vi "laneleftright412_temp.vi"() -> ()   [LabVIEW 2015]
uses:
  <vilib>/Analysis/1siggen.llb/Ramp Pattern by Delta.vi
  G_ALL.vi
  <vilib>/Analysis/polynomials.llb/nth Derivative of Polynomial (DBL).vi
  <vilib>/Analysis/polynomials.llb/Scalar Polynomial Evaluation (DBL).vi
  G_LCM.vi
  G_SEN.vi
  <vilib>/Analysis/NI_AALBase.lvlib
  <vilib>/Analysis/NI_AALPro.lvlib
panel:
  out "size(s)":i32
  out "lf_shift":dbl
  out "lr_shift":dbl
  out "rf_shift":dbl
  out "rr_shift":dbl
  in  "gain":dbl=1.0
  out "y_shift":dbl format="%#_13g"
  out "x_shift":dbl format="%#_13g"
  in  "d_safe":dbl=0.4
  out "R0":dbl
  out "y_ramp":dbl[](array[numeric])
  out "y_car":dbl[](array[numeric])
  out "x_car":dbl[](array[numeric])
  out "x_rf":dbl[](array[numeric])
  out "y_rf":dbl[](array[numeric])
  out "y_rr":dbl[](array[numeric])
  out "x_rr":dbl[](array[numeric])
  out "x_lr":dbl[](array[numeric])
  out "y_lr":dbl[](array[numeric])
  out "af":dbl
  out "y_lf":dbl[](array[numeric])
  out "x_lf":dbl[](array[numeric])
  out "h_path":dbl[](array[numeric])
  out "x_path":dbl[](array[numeric])
  out "y_path":dbl[](array[numeric])
  out "gap":dbl
  out "theta":dbl[](array[numeric])
  out "y":dbl[](array[numeric])
  out "x":dbl[](array[numeric])
  out "r":dbl[](array[numeric])
  out "rout":dbl[](array[numeric])
  out "rin":dbl[](array[numeric])
  out "XY Graph":cluster{"Y":dbl[], "Y":dbl[]}[](graph)
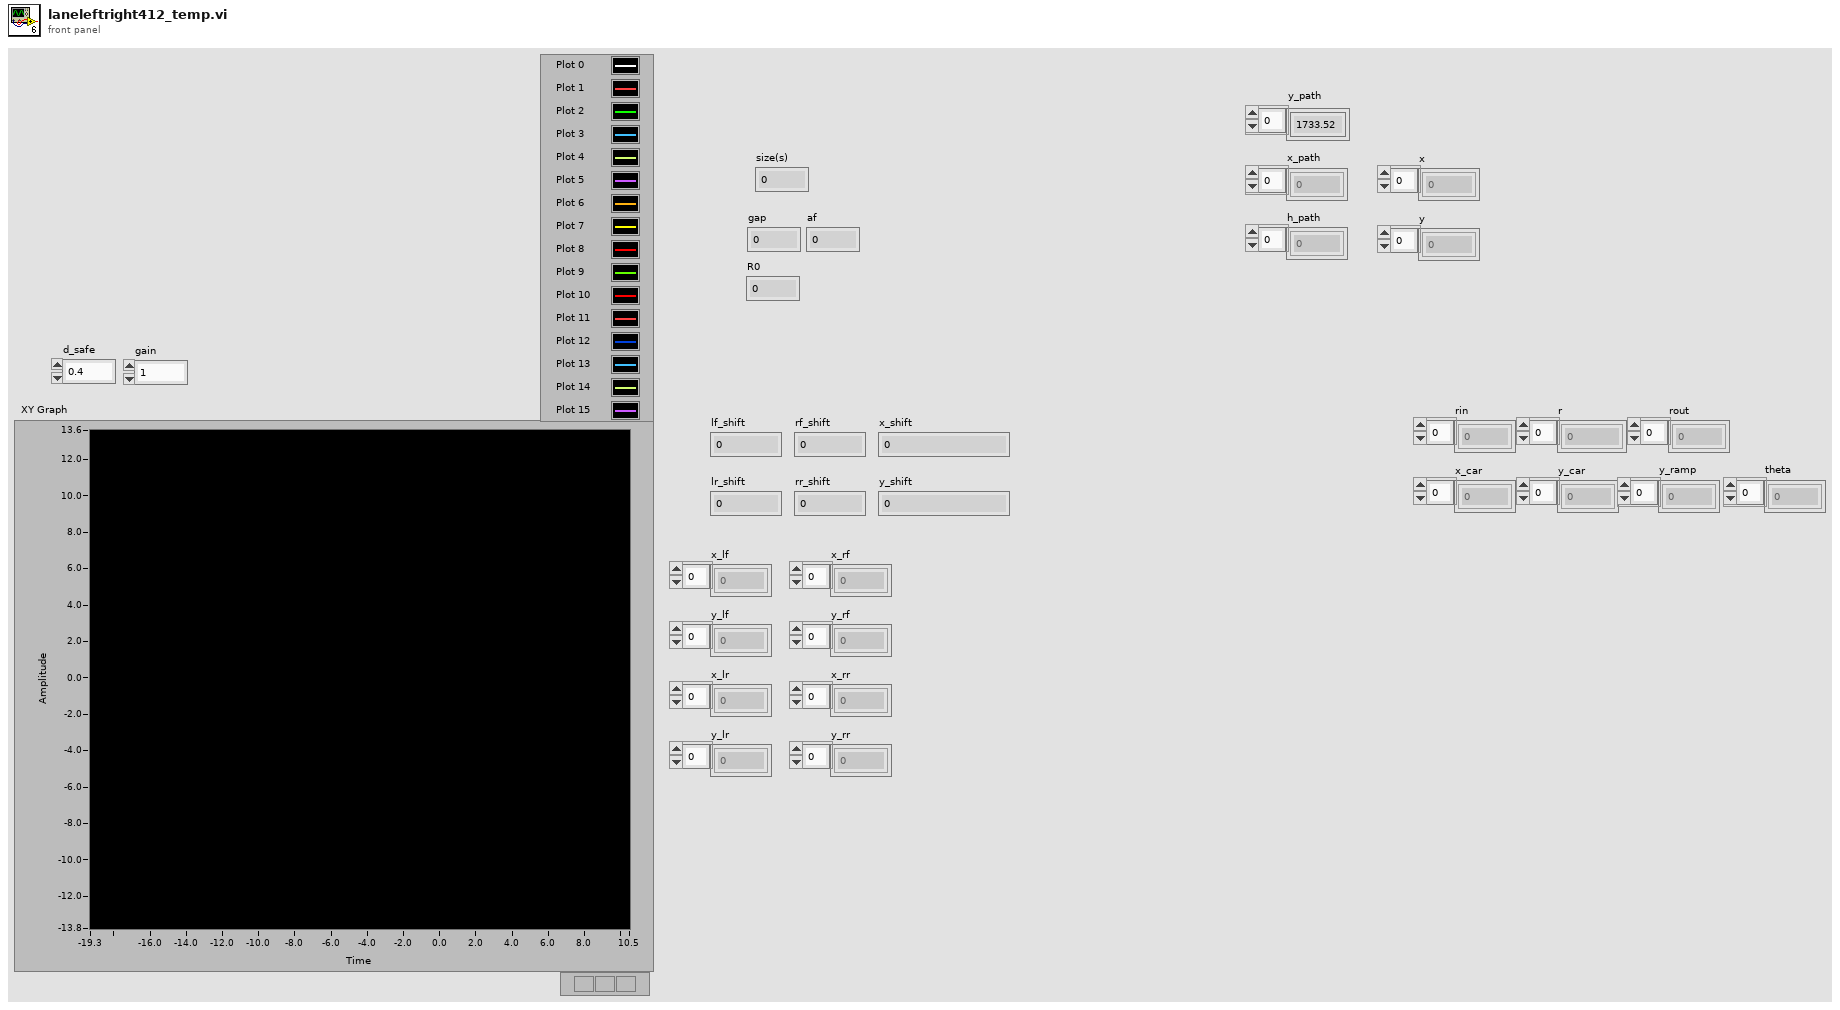
[diagram p1: front panel]
types:
  T1 = cluster{"C_Wheel base":dbl, "ratio_steer":dbl, "Overall width":dbl, "af":dbl, "turn radius":dbl, "eval":dbl, "ap":dbl, "an":dbl, "Vmax":dbl, "mu":dbl, "Vlast":dbl}
  T2 = cluster{"hash":i64, "sys time":i64, "size":i64, "x":dbl[], "y":dbl[], "point_flag":i32[]}
  T3 = cluster{"delta":bool, "Rotational position":dbl, "Rotational position":dbl}[]
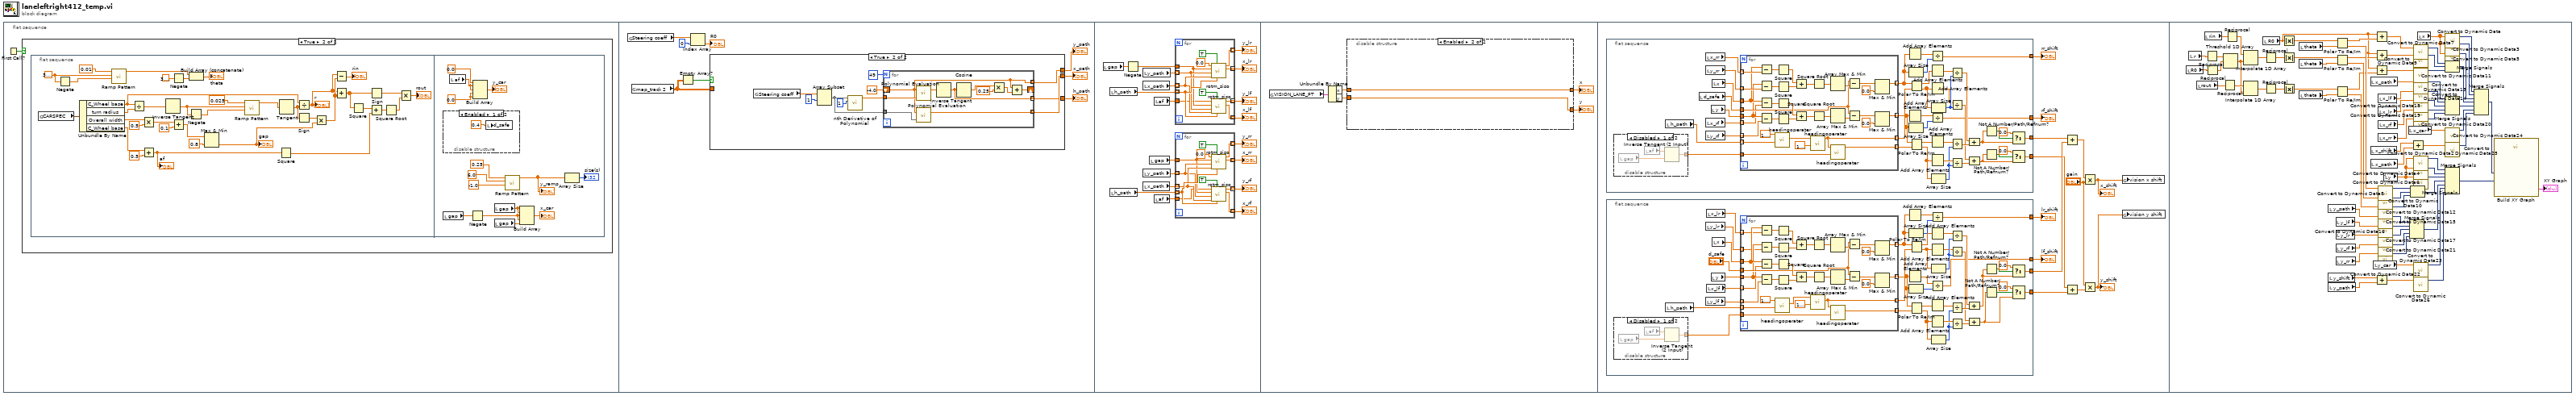
[diagram p0: block diagram]
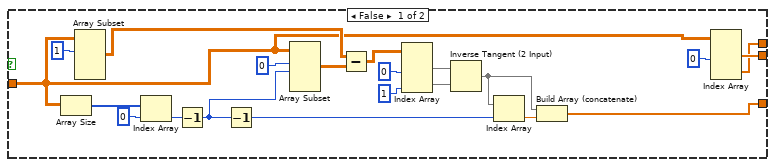
[diagram p4: hidden frame]
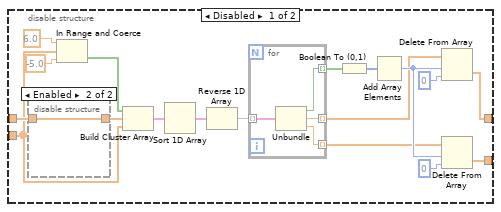
[diagram p5: hidden frame]
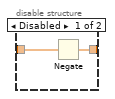
[diagram p6: hidden frame]
diagram:
  n1 = flat-sequence {
    frame #0 {
      n2 = First Call?() -> (First Call?: T/F=w1:bool)
      n3 = case shown="True" w1 {
        frame False {
        }
        frame True {
          n4 = flat-sequence {
            frame #0 {
              w20 = 3.141592653589793
              n5 = global read "G_ALL.vi" "CARSPEC"() -> (w38:T1)
              n6 = Negate(x=w20) -> (-x=w21:dbl)
              n7 = Unbundle By Name(w38) -> ("C_Wheel base"=w18:dbl, "turn radius"=w37:dbl, "Overall width"=w32:dbl, "C_Wheel base"=w4:dbl)
              n8 = call-poly <vilib>:"Ramp Pattern.vi"("start"=w21, "end"=w20, "delta"=0.01) -> ("Ramp Pattern"=w15:dbl[])  [unwired: 6 in, 2 out]
              n9 = Divide(x=w18, y=w37) -> (x/y=w36:dbl)
              n10 = Multiply(x=w32, y=0.5) -> (x*y=w17:dbl)
              n11 = Add(x=w4, y=0.5) -> (x+y=w2:dbl)
              "af" <- w2
              n12 = Inverse Tangent(1:w36) -> (0:w35:dbl)
              n13 = Negate(x=3.141592653589793) -> (-x=w12:dbl)
              n14 = Add(x=w17, y=0.1) -> (x+y=w7:dbl)
              n15 = Negate(x=w35) -> (-x=w8:dbl)
              n16 = Build Array (concatenate)(w15, w12) -> (→"theta":dbl[])
              n17 = Max & Min(x=w7, y=0.8) -> (min(x,y)=w6:dbl)  [unwired: 1 out]
              "gap" <- w6
              n18 = call-poly <vilib>:"Ramp Pattern.vi"("start"=w8, "end"=w35, "delta"=0.025) -> ("Ramp Pattern"=w33:dbl[])  [unwired: 6 in, 2 out]
              n19 = Square(x=w2) -> (x^2=w26:dbl)
              n20 = Tangent(1:w33) -> (0:w30:dbl[])
              n21 = Divide(x=w18, y=w30) -> (x/y=w11:dbl[])
              "r" <- w11
              n22 = Sign(1:w30) -> (0:w29:dbl[])
              n23 = Multiply(x=w29, y=w6) -> (x*y=w28:dbl[])
              n24 = Subtract(x=w11, y=w28) -> (x-y=→"rin":dbl[])
              n25 = Add(x=w11, y=w28) -> (x+y=w24:dbl[])
              n26 = Square(x=w24) -> (x^2=w27:dbl[])
              n27 = Sign(1:w24) -> (0:w22:dbl[])
              n28 = Add(x=w27, y=w26) -> (x+y=w25:dbl[])
              n29 = Square Root(x=w25) -> (sqrt(x)=w23:dbl[])
              n30 = Multiply(x=w22, y=w23) -> (x*y=→"rout":dbl[])
            }
            frame #1 {
              w45 = 0.0 ("element")
              n31 = disable-structure shown="Enabled" {
                frame Enabled {
                  n32 = local write "d_safe"(0.4 ("d_safe")) -> ()
                }
                frame Disabled {
                }
              }
              n33 = local read "gap"() -> (w52:dbl)
              n34 = local read "af"() -> (w47:dbl)
              n35 = Negate(x=w52) -> (-x=w50:dbl)
              n36 = Build Array(0.0 ("element"), w47, w47, w45, w45) -> (→"y_car":dbl[])
              n37 = local read "gap"() -> (w51:dbl)
              n38 = local read "gap"() -> (w49:dbl)
              n39 = call-poly <vilib>:"Ramp Pattern.vi"("start"=-1.0, "end"=6.0, "delta"=0.25) -> ("Ramp Pattern"=w40:dbl[])  [unwired: 6 in, 2 out]
              "y_ramp" <- w40
              n40 = Build Array(w51, w51, w50, w50, w49) -> (→"x_car":dbl[])
              n41 = Array Size(array=w40) -> (size(s)=→"size(s)":i32)
            }
          }
        }
      }
    }
    frame #1 {
      n42 = global read "G_ALL.vi" "Steering coeff"() -> (w58:dbl[])
      n43 = global read "G_ALL.vi" "map_track 2"() -> (w54:dbl[][])
      n44 = Empty Array?(array=w54) -> (empty?=w55:bool)
      n45 = Index Array(array=w58, index=0) -> (element=→"R0":dbl)
      n46 = case shown="True" w55 {
        tunnel: [w82 w92] -> w61
        tunnel: [w81 w90] -> w60
        tunnel: [w80 w91] -> w59
        tunnel: w54 -> [w62 _]
        frame False {
          n47 = Array Size(array=w62) -> (size(s)=w77:i32[])
          n48 = Array Subset(array=w62, index (row)=1 ("index")) -> (w73:dbl[][])  [unwired: 3 in]
          n49 = Index Array(array=w77, index=0) -> (element=w75:i32)
          n50 = Decrement(x=w75) -> (x-1=w67:i32)
          n51 = Decrement(x=w67) -> (x-1=w66:i32)
          n52 = Array Subset(array=w62, index (row)=0 ("index"), length (row)=w67) -> (w74:dbl[][])  [unwired: 2 in]
          n53 = Subtract(x=w73, y=w74) -> (x-y=w72:dbl[][])
          n54 = Index Array(array=w72, index (col) #1=0 ("disabled index (col)"), index (col) #2=1 ("index (col)")) -> (element #1=w69:dbl[], element #2=w68:dbl[])  [unwired: 2 in]
          n55 = Inverse Tangent (2 Input)(1:w68, 2:w69) -> (0:w64:dbl[])
          n56 = Index Array(array=w64, index=w66) -> (element=w65:dbl)
          n57 = Build Array (concatenate)(w64, w65) -> (w81:dbl[])
          n58 = Index Array(array=w62, index (col) #1=0 ("disabled index (col)")) -> (element #1=w82:dbl[], element #2=w80:dbl[])  [unwired: 3 in]
        }
        frame True {
          n59 = global read "G_ALL.vi" "Steering coeff"() -> (w83:dbl[])
          n60 = Array Subset(array=w83, index=1) -> (w85:dbl[])  [unwired: 1 in]
          n61 = call-poly <vilib>:"nth Derivative of Polynomial.vi"("order"=1, "P(x)"=w85) -> ("Nth Derivative of P(x)"=w86:dbl[])  [unwired: 8 in, 1 out]
          n62 = for {
            N: 49 -> [_]
            shift-right: [w93] -> _
            shift-left: -4.0 -> [w94]
            tunnel: w86 -> [w102]
            tunnel: w85 -> [w98]
            tunnel: [w97] -> w92 mode=indexing
            tunnel: [w94] -> w91 mode=indexing
            tunnel: [w96] -> w90 mode=indexing
            n63 = call-poly <vilib>:"Polynomial Evaluation.vi"("P(x)"=w102, "a"=w94) -> ("P(a)"=w101:dbl)  [unwired: 1 out]
            n64 = call-poly <vilib>:"Polynomial Evaluation.vi"("P(x)"=w98, "a"=w94) -> ("P(a)"=w97:dbl)  [unwired: 1 out]
            n65 = Inverse Tangent(1:w101) -> (0:w96:dbl)
            n66 = Cosine(x=w96) -> (cos(x)=w100:dbl)
            n67 = Multiply(x=w100, y=0.25) -> (x*y=w95:dbl)
            n68 = Add(x=w94, y=w95) -> (x+y=w93:dbl)
          }
        }
      }
      "y_path" <- w59
      "x_path" <- w61
      "h_path" <- w60
    }
    frame #2 {
      n69 = local read "gap"() -> (w118:dbl)
      n70 = local read "h_path"() -> (w119:dbl[])
      n71 = local read "h_path"() -> (w108:dbl[])
      n72 = Negate(x=w118) -> (-x=w117:dbl)
      n73 = local read "y_path"() -> (w120:dbl[])
      n74 = local read "x_path"() -> (w121:dbl[])
      n75 = local read "y_path"() -> (w107:dbl[])
      n76 = local read "x_path"() -> (w106:dbl[])
      n77 = local read "gap"() -> (w105:dbl)
      n78 = local read "af"() -> (w104:dbl)
      n79 = local read "af"() -> (w103:dbl)
      n80 = for {
        tunnel: w121 -> [w141] mode=indexing
        tunnel: w120 -> [w140] mode=indexing
        tunnel: w119 -> [w142] mode=indexing
        tunnel: [w145] -> w116 mode=indexing
        tunnel: [w144] -> w115 mode=indexing
        tunnel: w117 -> [w139]
        tunnel: [w137] -> w114 mode=indexing
        tunnel: [w136] -> w113 mode=indexing
        tunnel: w104 -> [w134]
        n81 = call "rotm_siso.vi"("angle[rad]"=w142, "reverse"=TRUE, "y0"=w141, "x0"=w140, "y"=w139, "x"=0.0) -> ("y'"=w136:dbl, "x'"=w137:dbl)  [unwired: 4 in]
        n82 = call "rotm_siso.vi"("angle[rad]"=w142, "reverse"=TRUE, "y0"=w141, "x0"=w140, "y"=w139, "x"=w134) -> ("y'"=w144:dbl, "x'"=w145:dbl)  [unwired: 4 in]
      }
      "x_lf" <- w115
      "y_lf" <- w116
      "y_lr" <- w114
      "x_lr" <- w113
      n83 = for {
        tunnel: w106 -> [w129] mode=indexing
        tunnel: w107 -> [w128] mode=indexing
        tunnel: w108 -> [w130] mode=indexing
        tunnel: [w133] -> w109 mode=indexing
        tunnel: [w132] -> w110 mode=indexing
        tunnel: w105 -> [w123]
        tunnel: [w126] -> w111 mode=indexing
        tunnel: [w125] -> w112 mode=indexing
        tunnel: w103 -> [w122]
        n84 = call "rotm_siso.vi"("angle[rad]"=w130, "reverse"=TRUE, "y0"=w129, "x0"=w128, "y"=w123, "x"=0.0) -> ("y'"=w125:dbl, "x'"=w126:dbl)  [unwired: 4 in]
        n85 = call "rotm_siso.vi"("angle[rad]"=w130, "reverse"=TRUE, "y0"=w129, "x0"=w128, "y"=w123, "x"=w122) -> ("y'"=w132:dbl, "x'"=w133:dbl)  [unwired: 4 in]
      }
      "x_rf" <- w110
      "y_rf" <- w109
      "y_rr" <- w111
      "x_rr" <- w112
    }
    frame #3 {
      n86 = global read "G_LCM.vi" "VISION_LANE_PT"() -> (w150:T2)
      n87 = Unbundle By Name(w150) -> ("x"=w149:dbl[], "y"=w148:dbl[])
      n88 = disable-structure shown="Enabled" {
        disable-tunnel: w149 -> [w167 w177]
        disable-tunnel: [w165 w176] -> w146
        disable-tunnel: [w164 w177] -> w147
        disable-tunnel: w148 -> [w161 w176]
        frame Disabled {
          n89 = disable-structure shown="Enabled" {
            disable-tunnel: w167 -> [w170 w171]
            disable-tunnel: [w169 w171] -> w168
            frame Disabled {
              n90 = Negate(x=w170) -> (-x=w169:dbl[])
            }
            frame Enabled {
            }
          }
          n91 = In Range and Coerce(upper limit=6.0 ("delta"), x=w161, lower limit=-5.0) -> (In Range?=w159:bool[])  [unwired: 1 out]
          n92 = Build Cluster Array(w159, w168, w161) -> (w157:T3)
          n93 = Sort 1D Array(array=w157) -> (sorted array=w158:T3)
          n94 = Reverse 1D Array(array=w158) -> (reversed array=w154:T3)
          n95 = for {
            tunnel: w154 -> [w175] mode=indexing
            tunnel: [w174] -> w152 mode=indexing
            tunnel: [w173] -> w151 mode=indexing
            tunnel: [w172] -> w162 mode=indexing
            n96 = Unbundle(w175) -> ("delta"=w172:bool, "Rotational position"=w174:dbl, "Rotational position"=w173:dbl)
          }
          n97 = Boolean To (0,1)(Boolean=w162) -> (0, 1=w155:i16[])
          n98 = Add Array Elements(numeric array=w155) -> (sum=w163:i16)
          n99 = Delete From Array(array=w152, length=w163, index=0) -> (deleted portion=w164:dbl[])  [unwired: 1 out]
          n100 = Delete From Array(array=w151, length=w163, index=0) -> (deleted portion=w165:dbl[])  [unwired: 1 out]
        }
        frame Enabled {
        }
      }
      "x" <- w147
      "y" <- w146
    }
    frame #4 {
      n101 = flat-sequence {
        tunnel: [w203] -> w180
        tunnel: [w202] -> w183
        tunnel: [w196] -> w185
        tunnel: [w195] -> w184
        frame #0 {
          n102 = disable-structure shown="Disabled" {
            disable-tunnel: [w233 _] -> w194
            frame Disabled {
              n103 = local read "gap"() -> (w234:dbl)
              n104 = local read "af"() -> (w232:dbl)
              n105 = Inverse Tangent (2 Input)(1:w234, 2:w232) -> (0:w233:dbl)
            }
            frame Enabled {
            }
          }
          n106 = local read "h_path"() -> (w227:dbl[])
          n107 = local read "d_safe"() -> (w191:dbl)
          n108 = local read "x_rr"() -> (w226:dbl[])
          n109 = local read "y_rr"() -> (w225:dbl[])
          n110 = local read "x_rf"() -> (w228:dbl[])
          n111 = local read "y_rf"() -> (w229:dbl[])
          n112 = local read "y"() -> (w230:dbl[])
          n113 = local read "x"() -> (w231:dbl[])
          n114 = for {
            tunnel: w231 -> [w245]
            tunnel: w230 -> [w244]
            tunnel: w229 -> [w268] mode=indexing
            tunnel: w228 -> [w240] mode=indexing
            tunnel: w227 -> [w242] mode=indexing
            tunnel: [w236] -> w224 mode=indexing
            tunnel: w191 -> [w246]
            tunnel: [w259] -> w192 mode=indexing
            tunnel: [w258] -> w199 mode=indexing
            tunnel: w226 -> [w248] mode=indexing
            tunnel: w225 -> [w247] mode=indexing
            tunnel: w194 -> [w235]
            tunnel: [w237] -> w193 mode=indexing
            n115 = Subtract(x=w245, y=w248) -> (x-y=w249:dbl[])
            n116 = Subtract(x=w244, y=w247) -> (x-y=w250:dbl[])
            n117 = Subtract(x=w245, y=w240) -> (x-y=w267:dbl[])
            n118 = Subtract(x=w244, y=w268) -> (x-y=w266:dbl[])
            n119 = call "headingoperater.vi"("h1"=w242, "h2"=1.5707963267948966) -> ("h2-h1"=w241:dbl)  [unwired: 8 in, 1 out]
            n120 = Square(x=w249) -> (x^2=w252:dbl[])
            n121 = Square(x=w250) -> (x^2=w251:dbl[])
            n122 = Square(x=w267) -> (x^2=w264:dbl[])
            n123 = Square(x=w266) -> (x^2=w265:dbl[])
            n124 = Add(x=w252, y=w251) -> (x+y=w253:dbl[])
            n125 = Add(x=w264, y=w265) -> (x+y=w263:dbl[])
            n126 = call "headingoperater.vi"("h1"=1.5707963267948966, "h2"=w241) -> ("h2+h1"=w236:dbl)  [unwired: 8 in, 1 out]
            n127 = Square Root(x=w253) -> (sqrt(x)=w254:dbl[])
            n128 = Square Root(x=w263) -> (sqrt(x)=w262:dbl[])
            n129 = Array Max & Min(array=w254) -> (min value=w255:dbl)  [unwired: 3 out]
            n130 = Array Max & Min(array=w262) -> (min value=w239:dbl)  [unwired: 3 out]
            n131 = call "headingoperater.vi"("h1"=w235, "h2"=w236) -> ("h2+h1"=w237:dbl)  [unwired: 8 in, 1 out]
            n132 = Subtract(x=w246, y=w255) -> (x-y=w256:dbl)
            n133 = Subtract(x=w246, y=w239) -> (x-y=w238:dbl)
            n134 = Max & Min(x=w256, y=0.0) -> (max(x,y)=w258:dbl)  [unwired: 1 out]
            n135 = Max & Min(x=w238, y=0.0) -> (max(x,y)=w259:dbl)  [unwired: 1 out]
          }
          n136 = Add Array Elements(numeric array=w199) -> (sum=w201:dbl)
          n137 = Add Array Elements(numeric array=w192) -> (sum=w197:dbl)
          n138 = Array Size(array=w199) -> (size(s)=w200:i32)
          n139 = Array Size(array=w192) -> (size(s)=w198:i32)
          n140 = Polar To Re/Im(2:w224, 3:w199) -> (0:w219:dbl[], 1:w220:dbl[])
          n141 = Polar To Re/Im(2:w193, 3:w192) -> (0:w214:dbl[], 1:w215:dbl[])
          n142 = Divide(x=w201, y=w200) -> (x/y=w196:dbl)
          n143 = Add Array Elements(numeric array=w220) -> (sum=w222:dbl)
          n144 = Add Array Elements(numeric array=w219) -> (sum=w221:dbl)
          n145 = Divide(x=w197, y=w198) -> (x/y=w195:dbl)
          n146 = Add Array Elements(numeric array=w215) -> (sum=w217:dbl)
          n147 = Add Array Elements(numeric array=w214) -> (sum=w218:dbl)
          n148 = Array Size(array=w219) -> (size(s)=w223:i32)
          n149 = Array Size(array=w214) -> (size(s)=w216:i32)
          n150 = Divide(x=w222, y=w223) -> (x/y=w213:dbl)
          n151 = Divide(x=w221, y=w223) -> (x/y=w211:dbl)
          n152 = Divide(x=w217, y=w216) -> (x/y=w212:dbl)
          n153 = Divide(x=w218, y=w216) -> (x/y=w210:dbl)
          n154 = Compound Arithmetic op=ADD(w213, w212) -> (w207:dbl)
          n155 = Compound Arithmetic op=ADD(w211, w210) -> (w204:dbl)
          n156 = Not A Number/Path/Refnum?(number/path/refnum=w207) -> (NaN/Path/Refnum?=w208:bool)
          n157 = Not A Number/Path/Refnum?(number/path/refnum=w204) -> (NaN/Path/Refnum?=w206:bool)
          n158 = Select(t=0.0, s=w208, f=w207) -> (s? t:f=w202:dbl)
          n159 = Select(t=0.0, s=w206, f=w204) -> (s? t:f=w203:dbl)
        }
      }
      n160 = flat-sequence {
        tunnel: [w280] -> w179
        tunnel: [w279] -> w182
        tunnel: [w272] -> w188
        tunnel: [w271] -> w187
        frame #0 {
          n161 = disable-structure shown="Disabled" {
            disable-tunnel: [w311 _] -> w270
            frame Disabled {
              n162 = local read "gap"() -> (w312:dbl)
              n163 = local read "af"() -> (w310:dbl)
              n164 = Inverse Tangent (2 Input)(1:w312, 2:w310) -> (0:w311:dbl)
            }
            frame Enabled {
            }
          }
          n165 = local read "h_path"() -> (w307:dbl[])
          n166 = local read "y_lr"() -> (w303:dbl[])
          n167 = local read "y_lf"() -> (w301:dbl[])
          n168 = local read "x_lr"() -> (w304:dbl[])
          n169 = local read "x_lf"() -> (w302:dbl[])
          n170 = local read "y"() -> (w308:dbl[])
          n171 = local read "x"() -> (w309:dbl[])
          n172 = for {
            tunnel: w309 -> [w324]
            tunnel: w308 -> [w323]
            tunnel: w307 -> [w317] mode=indexing
            tunnel: "d_safe" -> [w325]
            tunnel: [w315] -> w305 mode=indexing
            tunnel: [w336] -> w273 mode=indexing
            tunnel: [w337] -> w276 mode=indexing
            tunnel: w304 -> [w322] mode=indexing
            tunnel: w303 -> [w321] mode=indexing
            tunnel: w302 -> [w320] mode=indexing
            tunnel: w301 -> [w319] mode=indexing
            tunnel: w270 -> [w313]
            tunnel: [w314] -> w269 mode=indexing
            n173 = Subtract(x=w324, y=w322) -> (x-y=w346:dbl[])
            n174 = Subtract(x=w323, y=w321) -> (x-y=w345:dbl[])
            n175 = Subtract(x=w324, y=w320) -> (x-y=w326:dbl[])
            n176 = Subtract(x=w323, y=w319) -> (x-y=w327:dbl[])
            n177 = call "headingoperater.vi"("h1"=w317, "h2"=1.5707963267948966) -> ("h2-h1"=w316:dbl)  [unwired: 8 in, 1 out]
            n178 = Square(x=w346) -> (x^2=w343:dbl[])
            n179 = Square(x=w345) -> (x^2=w344:dbl[])
            n180 = Square(x=w326) -> (x^2=w329:dbl[])
            n181 = Square(x=w327) -> (x^2=w328:dbl[])
            n182 = Add(x=w343, y=w344) -> (x+y=w342:dbl[])
            n183 = Add(x=w329, y=w328) -> (x+y=w330:dbl[])
            n184 = call "headingoperater.vi"("h1"=1.5707963267948966, "h2"=w316) -> ("h2-h1"=w315:dbl)  [unwired: 8 in, 1 out]
            n185 = Square Root(x=w342) -> (sqrt(x)=w341:dbl[])
            n186 = Square Root(x=w330) -> (sqrt(x)=w331:dbl[])
            n187 = Array Max & Min(array=w341) -> (min value=w340:dbl)  [unwired: 3 out]
            n188 = Array Max & Min(array=w331) -> (min value=w333:dbl)  [unwired: 3 out]
            n189 = call "headingoperater.vi"("h1"=w313, "h2"=w315) -> ("h2-h1"=w314:dbl)  [unwired: 8 in, 1 out]
            n190 = Subtract(x=w325, y=w340) -> (x-y=w339:dbl)
            n191 = Subtract(x=w325, y=w333) -> (x-y=w334:dbl)
            n192 = Max & Min(x=w339, y=0.0) -> (max(x,y)=w337:dbl)  [unwired: 1 out]
            n193 = Max & Min(x=w334, y=0.0) -> (max(x,y)=w336:dbl)  [unwired: 1 out]
          }
          n194 = Add Array Elements(numeric array=w276) -> (sum=w277:dbl)
          n195 = Add Array Elements(numeric array=w273) -> (sum=w275:dbl)
          n196 = Array Size(array=w276) -> (size(s)=w278:i32)
          n197 = Array Size(array=w273) -> (size(s)=w274:i32)
          n198 = Polar To Re/Im(2:w305, 3:w276) -> (0:w296:dbl[], 1:w297:dbl[])
          n199 = Polar To Re/Im(2:w269, 3:w273) -> (0:w291:dbl[], 1:w292:dbl[])
          n200 = Divide(x=w277, y=w278) -> (x/y=w272:dbl)
          n201 = Add Array Elements(numeric array=w297) -> (sum=w299:dbl)
          n202 = Add Array Elements(numeric array=w296) -> (sum=w298:dbl)
          n203 = Divide(x=w275, y=w274) -> (x/y=w271:dbl)
          n204 = Add Array Elements(numeric array=w292) -> (sum=w294:dbl)
          n205 = Add Array Elements(numeric array=w291) -> (sum=w295:dbl)
          n206 = Array Size(array=w296) -> (size(s)=w300:i32)
          n207 = Array Size(array=w291) -> (size(s)=w293:i32)
          n208 = Divide(x=w299, y=w300) -> (x/y=w290:dbl)
          n209 = Divide(x=w298, y=w300) -> (x/y=w288:dbl)
          n210 = Divide(x=w294, y=w293) -> (x/y=w289:dbl)
          n211 = Divide(x=w295, y=w293) -> (x/y=w287:dbl)
          n212 = Compound Arithmetic op=ADD(w290, w289) -> (w284:dbl)
          n213 = Compound Arithmetic op=ADD(w288, w287) -> (w281:dbl)
          n214 = Not A Number/Path/Refnum?(number/path/refnum=w284) -> (NaN/Path/Refnum?=w285:bool)
          n215 = Not A Number/Path/Refnum?(number/path/refnum=w281) -> (NaN/Path/Refnum?=w283:bool)
          n216 = Select(t=0.0, s=w285, f=w284) -> (s? t:f=w279:dbl)
          n217 = Select(t=0.0, s=w283, f=w281) -> (s? t:f=w280:dbl)
        }
      }
      n218 = Add(x=w183, y=w182) -> (x+y=w181:dbl)
      n219 = Add(x=w180, y=w179) -> (x+y=w178:dbl)
      n220 = Multiply(x=w181, y="gain") -> (x*y=w190:dbl)
      "x_shift" <- w190
      n221 = Multiply(x="gain", y=w178) -> (x*y=w189:dbl)
      "y_shift" <- w189
      n222 = global write "G_SEN.vi" "vision x shift"(w190) -> ()
      n223 = global write "G_SEN.vi" "vision y shift"(w189) -> ()
      "rr_shift" <- w185
      "rf_shift" <- w184
      "lr_shift" <- w188
      "lf_shift" <- w187
    }
    frame #5 {
      n224 = local read "R0"() -> (w372:dbl)
      n225 = local read "r"() -> (w371:dbl[])
      n226 = local read "rout"() -> (w362:dbl[])
      n227 = local read "rin"() -> (w368:dbl[])
      n228 = Reciprocal(x=w371) -> (1/x=w370:dbl[])
      n229 = Reciprocal(x=w372) -> (1/x=w369:dbl)
      n230 = Reciprocal(x=w362) -> (1/x=w363:dbl[])
      n231 = Threshold 1D Array(2:w369, 3:w370) -> (0:w361:dbl)  [unwired: 1 in]
      n232 = Reciprocal(x=w368) -> (1/x=w367:dbl[])
      n233 = Interpolate 1D Array(1:w361, 2:w367) -> (0:w366:dbl)
      n234 = Interpolate 1D Array(1:w361, 2:w363) -> (0:w364:dbl)
      n235 = local read "R0"() -> (w359:dbl)
      n236 = Reciprocal(x=w366) -> (1/x=w365:dbl)
      n237 = Reciprocal(x=w364) -> (1/x=w360:dbl)
      n238 = Absolute Value(x=w359) -> (abs(x)=w418:dbl)
      n239 = Absolute Value(x=w365) -> (abs(x)=w413:dbl)
      n240 = Absolute Value(x=w360) -> (abs(x)=w408:dbl)
      n241 = local read "theta"() -> (w419:dbl[])
      n242 = local read "theta"() -> (w412:dbl[])
      n243 = local read "theta"() -> (w409:dbl[])
      n244 = local read "y_path"() -> (w386:dbl[])
      n245 = local read "y_shift"() -> (w349:dbl)
      n246 = local read "y_path"() -> (w350:dbl[])
      n247 = Polar To Re/Im(2:w419, 3:w418) -> (0:w415:dbl[], 1:w417:dbl[])
      n248 = Polar To Re/Im(2:w412, 3:w413) -> (0:w410:dbl[], 1:w414:dbl[])
      n249 = Polar To Re/Im(2:w409, 3:w408) -> (0:w405:dbl[], 1:w407:dbl[])
      n250 = local read "y_lf"() -> (w392:dbl[])
      n251 = local read "y_lr"() -> (w385:dbl[])
      n252 = local read "y_rf"() -> (w379:dbl[])
      n253 = local read "y_rr"() -> (w380:dbl[])
      n254 = local read "x_path"() -> (w398:dbl[])
      n255 = local read "x_shift"() -> (w353:dbl)
      n256 = local read "x_path"() -> (w354:dbl[])
      n257 = local read "y_car"() -> (w376:dbl[])
      n258 = Add(x=w359, y=w417) -> (x+y=w416:dbl[])
      n259 = Add(x=w359, y=w414) -> (x+y=w411:dbl[])
      n260 = Add(x=w359, y=w407) -> (x+y=w406:dbl[])
      n261 = Add(x=w349, y=w350) -> (x+y=w348:dbl[])
      n262 = local read "x_lf"() -> (w396:dbl[])
      n263 = local read "x_lr"() -> (w388:dbl[])
      n264 = local read "x_rf"() -> (w383:dbl[])
      n265 = local read "x_rr"() -> (w384:dbl[])
      n266 = call "Convert to Dynamic Data8"("Array"=w415) -> ("Dynamic Data Type"=w401:dynamicdata)  [unwired: 3 in]
      n267 = call "Convert to Dynamic Data10"("Array"=w410) -> ("Dynamic Data Type"=w400:dynamicdata)  [unwired: 3 in]
      n268 = call "Convert to Dynamic Data12"("Array"=w405) -> ("Dynamic Data Type"=w399:dynamicdata)  [unwired: 3 in]
      n269 = call "Convert to Dynamic Data15"("Array"=w386) -> ("Dynamic Data Type"=w391:dynamicdata)  [unwired: 3 in]
      n270 = call "Convert to Dynamic Data16"("Array"=w392) -> ("Dynamic Data Type"=w393:dynamicdata)  [unwired: 3 in]
      n271 = call "Convert to Dynamic Data17"("Array"=w385) -> ("Dynamic Data Type"=w389:dynamicdata)  [unwired: 3 in]
      n272 = call "Convert to Dynamic Data21"("Array"=w379) -> ("Dynamic Data Type"=w378:dynamicdata)  [unwired: 3 in]
      n273 = call "Convert to Dynamic Data22"("Array"=w380) -> ("Dynamic Data Type"=w377:dynamicdata)  [unwired: 3 in]
      n274 = local read "y"() -> (w358:dbl[])
      n275 = local read "x_car"() -> (w374:dbl[])
      n276 = Merge Signals(w391, w393, w389, w378, w377) -> (w390:dynamicdata)
      n277 = Merge Signals(w401, w400, w399) -> (w355:dynamicdata)
      n278 = Add(x=w353, y=w354) -> (x+y=w352:dbl[])
      n279 = call "Convert to Dynamic Data7"("Array"=w416) -> ("Dynamic Data Type"=w404:dynamicdata)  [unwired: 3 in]
      n280 = call "Convert to Dynamic Data9"("Array"=w411) -> ("Dynamic Data Type"=w403:dynamicdata)  [unwired: 3 in]
      n281 = call "Convert to Dynamic Data11"("Array"=w406) -> ("Dynamic Data Type"=w402:dynamicdata)  [unwired: 3 in]
      n282 = call "Convert to Dynamic Data13"("Array"=w398) -> ("Dynamic Data Type"=w397:dynamicdata)  [unwired: 3 in]
      n283 = call "Convert to Dynamic Data14"("Array"=w396) -> ("Dynamic Data Type"=w395:dynamicdata)  [unwired: 3 in]
      n284 = call "Convert to Dynamic Data18"("Array"=w388) -> ("Dynamic Data Type"=w387:dynamicdata)  [unwired: 3 in]
      n285 = call "Convert to Dynamic Data19"("Array"=w383) -> ("Dynamic Data Type"=w382:dynamicdata)  [unwired: 3 in]
      n286 = call "Convert to Dynamic Data20"("Array"=w384) -> ("Dynamic Data Type"=w381:dynamicdata)  [unwired: 3 in]
      n287 = call "Convert to Dynamic Data2"("Array"=w358) -> ("Dynamic Data Type"=w428:dynamicdata)  [unwired: 3 in]
      n288 = call "Convert to Dynamic Data4"("Array"=w358) -> ("Dynamic Data Type"=w422:dynamicdata)  [unwired: 3 in]
      n289 = call "Convert to Dynamic Data6"("Array"=w358) -> ("Dynamic Data Type"=w420:dynamicdata)  [unwired: 3 in]
      n290 = call "Convert to Dynamic Data23"("Array"=w376) -> ("Dynamic Data Type"=w375:dynamicdata)  [unwired: 3 in]
      n291 = call "Convert to Dynamic Data26"("Array"=w348) -> ("Dynamic Data Type"=w347:dynamicdata)  [unwired: 3 in]
      n292 = local read "x"() -> (w357:dbl[])
      n293 = call "Convert to Dynamic Data"("Array"=w357) -> ("Dynamic Data Type"=w427:dynamicdata)  [unwired: 3 in]
      n294 = call "Convert to Dynamic Data3"("Array"=w357) -> ("Dynamic Data Type"=w424:dynamicdata)  [unwired: 3 in]
      n295 = call "Convert to Dynamic Data5"("Array"=w357) -> ("Dynamic Data Type"=w421:dynamicdata)  [unwired: 3 in]
      n296 = Merge Signals(w404, w403, w402) -> (w356:dynamicdata)
      n297 = Merge Signals(w397, w395, w387, w382, w381) -> (w394:dynamicdata)
      n298 = call "Convert to Dynamic Data24"("Array"=w374) -> ("Dynamic Data Type"=w373:dynamicdata)  [unwired: 3 in]
      n299 = call "Convert to Dynamic Data25"("Array"=w352) -> ("Dynamic Data Type"=w351:dynamicdata)  [unwired: 3 in]
      n300 = Merge Signals(w428, w422, w420, w355, w390, w375, w347) -> (w423:dynamicdata)
      n301 = Merge Signals(w427, w424, w421, w356, w394, w373, w351) -> (w425:dynamicdata)
      n302 = call "Build XY Graph"("Y Input"=w423, "X Input"=w425) -> ("XY Graph"=→"XY Graph":cluster{"X":dbl[], "Y":dbl[]}[])  [unwired: 8 in, 1 out]
    }
  }
